vi "matrix-test1.vi"() -> ()   [LabVIEW 2021]
uses:
  3-lorentzian-parameters.ctl
  <vilib>/Analysis/baseanly.llb/Matrix Type of Inverse Matrix.ctl
  <vilib>/Analysis/Matrix/Numeric/Conversions/Array To Matrix - RA2.vi
  <vilib>/Analysis/Matrix/Numeric/Conversions/Array To Matrix - RA.vi
  <vilib>/Analysis/7linalg.llb/Solve Linear Equations (multiple right hand).vi
  <vilib>/Analysis/Matrix/Numeric/Conversions/Matrix To Array - RM.vi
  <vilib>/Analysis/Matrix/NI_Matrix.lvlib
  <vilib>/Analysis/NI_AALBase.lvlib
  <vilib>/Analysis/NI_AALPro.lvlib
panel:
  out "Real 2D Array":dbl[][](array[numeric])
  out "parameters IN":map{T1, dbl}(c390)
  in  "Array 1":dbl[](array[numeric])
  in  "Array 2":dbl[][](array[numeric])
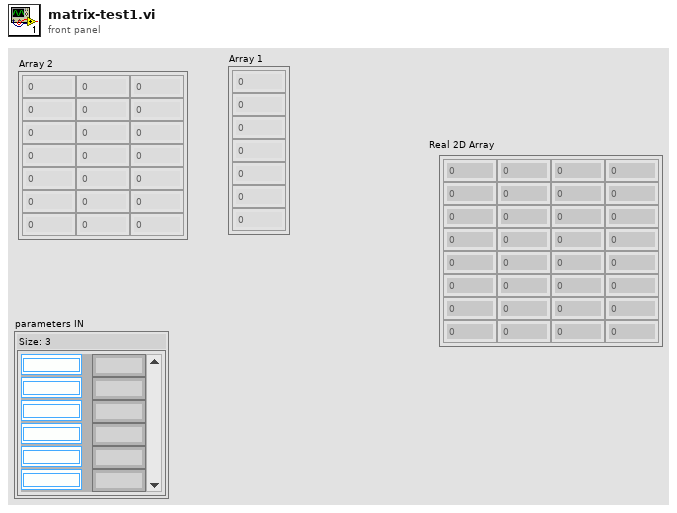
[diagram p1: front panel]
types:
  T1 = typedef "3-lorentzian-parameters.ctl" = enum16{"ζ", "τ1", "τS", "τN", "τC", "κ0", "m1", "m2", "m3", "T (K)", "B (T)", "θ (deg)", "side (S|R)", "set of (B|T)", "Re(offset)", "Im(offset)", "στ1", "στ1-", "στ1+", "στS", "στS-", "στS+", "στN", "στN-", "στN+", "τ11", "τ12", "τ21", "τ22", "τN1", "τN2"}
  T2 = typedef "NI_AALBase.lvlib/Matrix Type of Inverse Matrix.ctl" = enum32{"General", "Positive Definite", "Lower Triangular", "Upper Triangular"}
  T3 = typedef "NI_Matrix.lvlib/RealMatrix.ctl" = dbl[][]
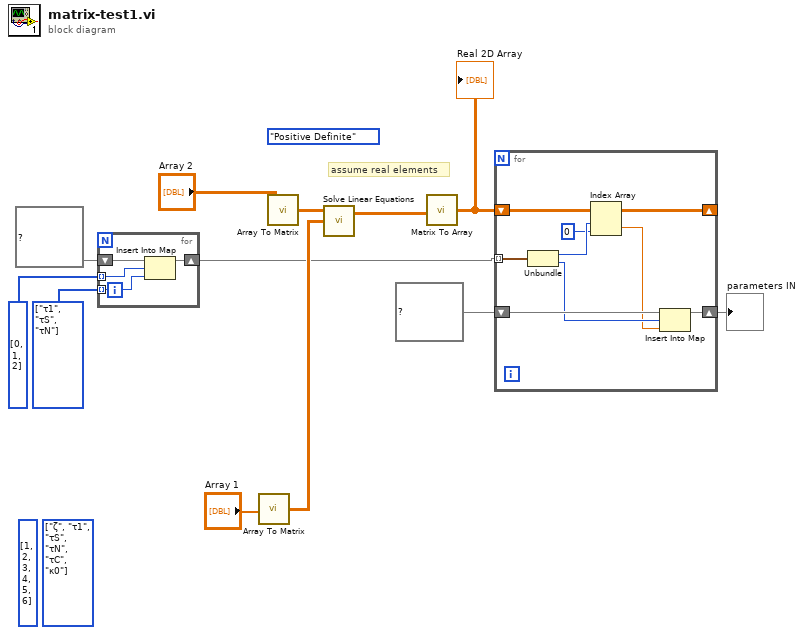
[diagram p0: block diagram]
diagram:
  (unwired) i32[] [1, 2, 3, 4, 5, 6]
  (unwired) T1[] [enum."ζ", enum."τ1", enum."τS", enum."τN", enum."τC", enum."κ0"] items=["ζ", "τ1", "τS", "τN", "τC", "κ0", "m1", "m2", "m3", "T (K)", "B (T)", "θ (deg)", "side (S|R)", "set of (B|T)", "Re(offset)", "Im(offset)", "στ1", "στ1-", "στ1+", "στS", "στS-", "στS+", "στN", "στN-", "στN+", "τ11", "τ12", "τ21", "τ22", "τN1", "τN2"]
  w5 = T1[] [enum."τ1", enum."τS", enum."τN"] items=["ζ", "τ1", "τS", "τN", "τC", "κ0", "m1", "m2", "m3", "T (K)", "B (T)", "θ (deg)", "side (S|R)", "set of (B|T)", "Re(offset)", "Im(offset)", "στ1", "στ1-", "στ1+", "στS", "στS-", "στS+", "στN", "στN-", "στN+", "τ11", "τ12", "τ21", "τ22", "τN1", "τN2"]
  (unwired) Matrix_Type_of_Inverse_Matrix."Positive Definite" ("matrix type")
  # "assume real elements"
  n1 = for {
    tunnel: w5 -> [w13] mode=indexing
    shift-right: [w15] -> w2
    shift-left: map{i32, T1} {} ("parameters IN") -> [w16]
    tunnel: i32[] [0, 1, 2] -> [w14] mode=indexing
    n2 = Insert Into Map(map in=w16, key=w14, value=w13) -> (map out=w15:map{i32, T1})  [unwired: 2 out]
  }
  n3 = call-poly <vilib>:"Array To Matrix.vi"("Real 1D Array"="Array 1") -> ("Real Matrix (Column Vector)"=w9:T3)
  n4 = call-poly <vilib>:"Array To Matrix.vi"("Real 2D Array"="Array 2") -> ("Real Matrix"=w10:T3)
  n5 = call-poly <vilib>:"Solve Linear Equations.vi"("Known Matrix"=w9, "Input Matrix"=w10) -> ("Solution Matrix"=w8:T3)  [unwired: 1 in, 1 out]
  n6 = call-poly <vilib>:"Matrix To Array.vi"("Real Matrix"=w8) -> ("Real 2D Array"=w12:dbl[][])
  "Real 2D Array" <- w12
  n7 = for {
    tunnel: w2 -> [w23] mode=indexing
    shift-right: [w24] -> _
    shift-left: w12 -> [w24]
    shift-right: [w21] -> w1
    shift-left: map{T1, dbl} {} ("parameters IN") -> [w22]
    n8 = Unbundle(w23) -> ("index"=w18:i32, "X selector"=w20:T1)
    n9 = Index Array(array=w24, index (row)=w18, index (col)=0 ("disabled index (col)")) -> (element=w19:dbl)
    n10 = Insert Into Map(map in=w22, key=w20, value=w19) -> (map out=w21:map{T1, dbl})  [unwired: 2 out]
  }
  "parameters IN" <- w1
